vi "Test Copy Active To All.vi"(8 "error in (no error)":errorcluster) -> (0 "error out":errorcluster)   [LabVIEW 2019]
uses:
  <vilib>/addons/_JKI Toolkits/Caraya/classes/Test/Test.lvclass
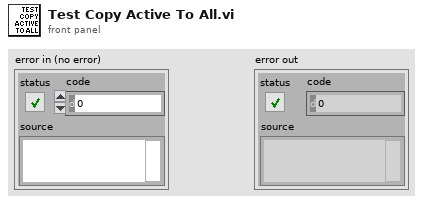
[diagram p1: front panel]
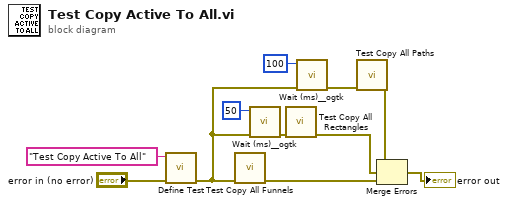
[diagram p0: block diagram]
diagram:
  n1 = call <vilib>:"Define Test.vi"("error in (no error)"="error in (no error)", "Label (VI Title)"="Test Copy Active To All") -> ("error out"=w7:errorcluster)  [unwired: 8 in, 1 out]
  n2 = call "Test Copy All Funnels.vi"("error in (no error)"=w7) -> ("error out"=w8:errorcluster)  [unwired: 10 in]
  n3 = call <userlib>:"Wait (ms)__ogtk.vi"("error in (no error)"=w7, "milliseconds to wait"=u32 50) -> ("error out"=w2:errorcluster)  [unwired: 8 in, 1 out]
  n4 = call "Test Copy All Rectangles.vi"("error in (no error)"=w2) -> ("error out"=w5:errorcluster)  [unwired: 10 in]
  n5 = call <userlib>:"Wait (ms)__ogtk.vi"("error in (no error)"=w7, "milliseconds to wait"=u32 100) -> ("error out"=w4:errorcluster)  [unwired: 8 in, 1 out]
  n6 = call "Test Copy All Paths.vi"("error in (no error)"=w4) -> ("error out"=w6:errorcluster)  [unwired: 10 in]
  n7 = Merge Errors(w6, w5, w8) -> (→"error out":errorcluster)
